vi "Unpack Boolean Value.vi"(11 "BooleanValueMsg in":refnum<class "BooleanValueMsg.lvclass">) -> (2 "Value":bool, 3 "Name":string)   [LabVIEW 2015, in "ActorAutoRegistration.lvlib" / "BooleanValueMsg.lvclass"]
uses:
  BooleanValueMsg.lvclass
  BooleanValueMsg.lvclass/BooleanValueMsg.ctl
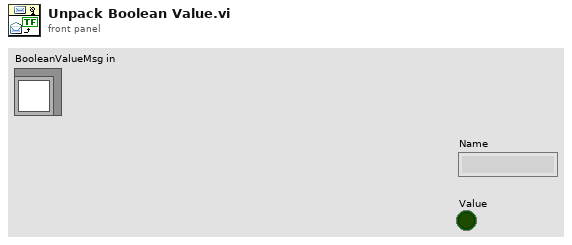
[diagram p1: front panel]
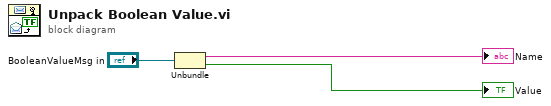
[diagram p0: block diagram]
diagram:
  n1 = Unbundle("BooleanValueMsg in") -> (→"Name":string, →"Value":bool)
